vi "TirfModule.vi"() -> ()   [LabVIEW 2012]
doc: "DESCRIPTION:\nThe One-Axis Move (Accel - Max Velocity - Decel) VI completes a move to user-specified position on a single axis while using user-specified acceleration, maximum velocity, and deceleration values. It also provides a monitor to track the progress of the move.\n\n*Note: This VI can be used as a subVI in a higher level program.\n\nINSTRUCTIONS:\n(1) Be sure your board is initialized before running this VI. Refer to the Initialization topic in the FlexMotion VI Online Help, which can be launched by choosing FlexMotion VI Online Help in the Help menu.\n\n(2) Select the Board ID that corresponds to your FlexMotion controller in the Board Configuration Utility. \n\n(3) Select the axis number to be used.\n\n(4) Set the Target Position (in encoder counts) to which you want the axis to move.\n\n(5) Set the values you wish to use for maximum velocity (RPM), acceleration (RPS/S), and deceleration (RPS/S).\n\n(6) Run the VI.\n\nKEY PARAMETERS:\n(1) Target Position: The position to which you want to move. This value needs to be changed every time you run the VI. If you run the VI twice in a row with the same target position, the motor will not move the second time since it will already be at its target position.\n\n(2) Velocity: The maximum velocity for the specified axis during the move.\n\n(3) Acceleration: The acceleration for the axis during the move.\n\n(4) Deceleration: The deceleration for the axis during the move. (This may be different than the acceleration.)\n\nI/O CONNECTIONS OVERVIEW:\nThis example requires a system configuration with one axis."
uses:
  MicroDrive.dll
panel:
  out "Found Epi":bool
  in  "Axis":u16(ring)=6 items=["1"=1, "2"=2, "3"=3, "4"=4, "5"=5, "6"=6]
  in  "Load":bool
  in  "Save":bool
  in  "clear5":bool
  in  "clear4":bool
  in  "clear3":bool
  in  "clear2":bool
  in  "clear1":bool
  in  "clear all":bool
  in  "write 5":bool
  in  "write 4":bool
  in  "write 3":bool
  in  "write 2":bool
  in  "write 1":bool
  in  "p4":bool
  in  "p5":bool
  in  "p3":bool
  in  "p2":bool
  in  "p1":bool
  out "Cluster":cluster{"Name":string[], "Position":dbl[]}
  out "Array 2":string[](array[string])
  out "Array":dbl[](array[numeric])
  out "Moving":bool
  in  "EPI":bool
  in  "Store":bool
  out "Current Position":dbl
  in  "Direction:":bool=TRUE
  out "Device Handle":i32
  in  "Velocity (mm/s)":dbl=1.0 min=0.01 max=2.0 format="%.3f"
  in  "Move size (µm)":dbl=50.0 format="%.3f"
  out "Forward Limit":bool
  out "Reverse Limit":bool
  in  "stop":bool
  in  "Move":bool
  # "Move To:"
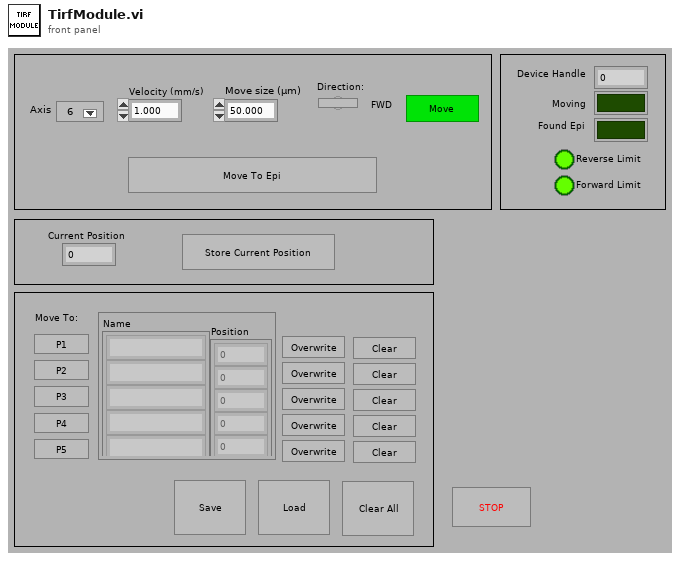
[diagram p1: front panel]
types:
  T1 = enum8{"Enabled", "Disabled", "Disabled and Grayed Out"}
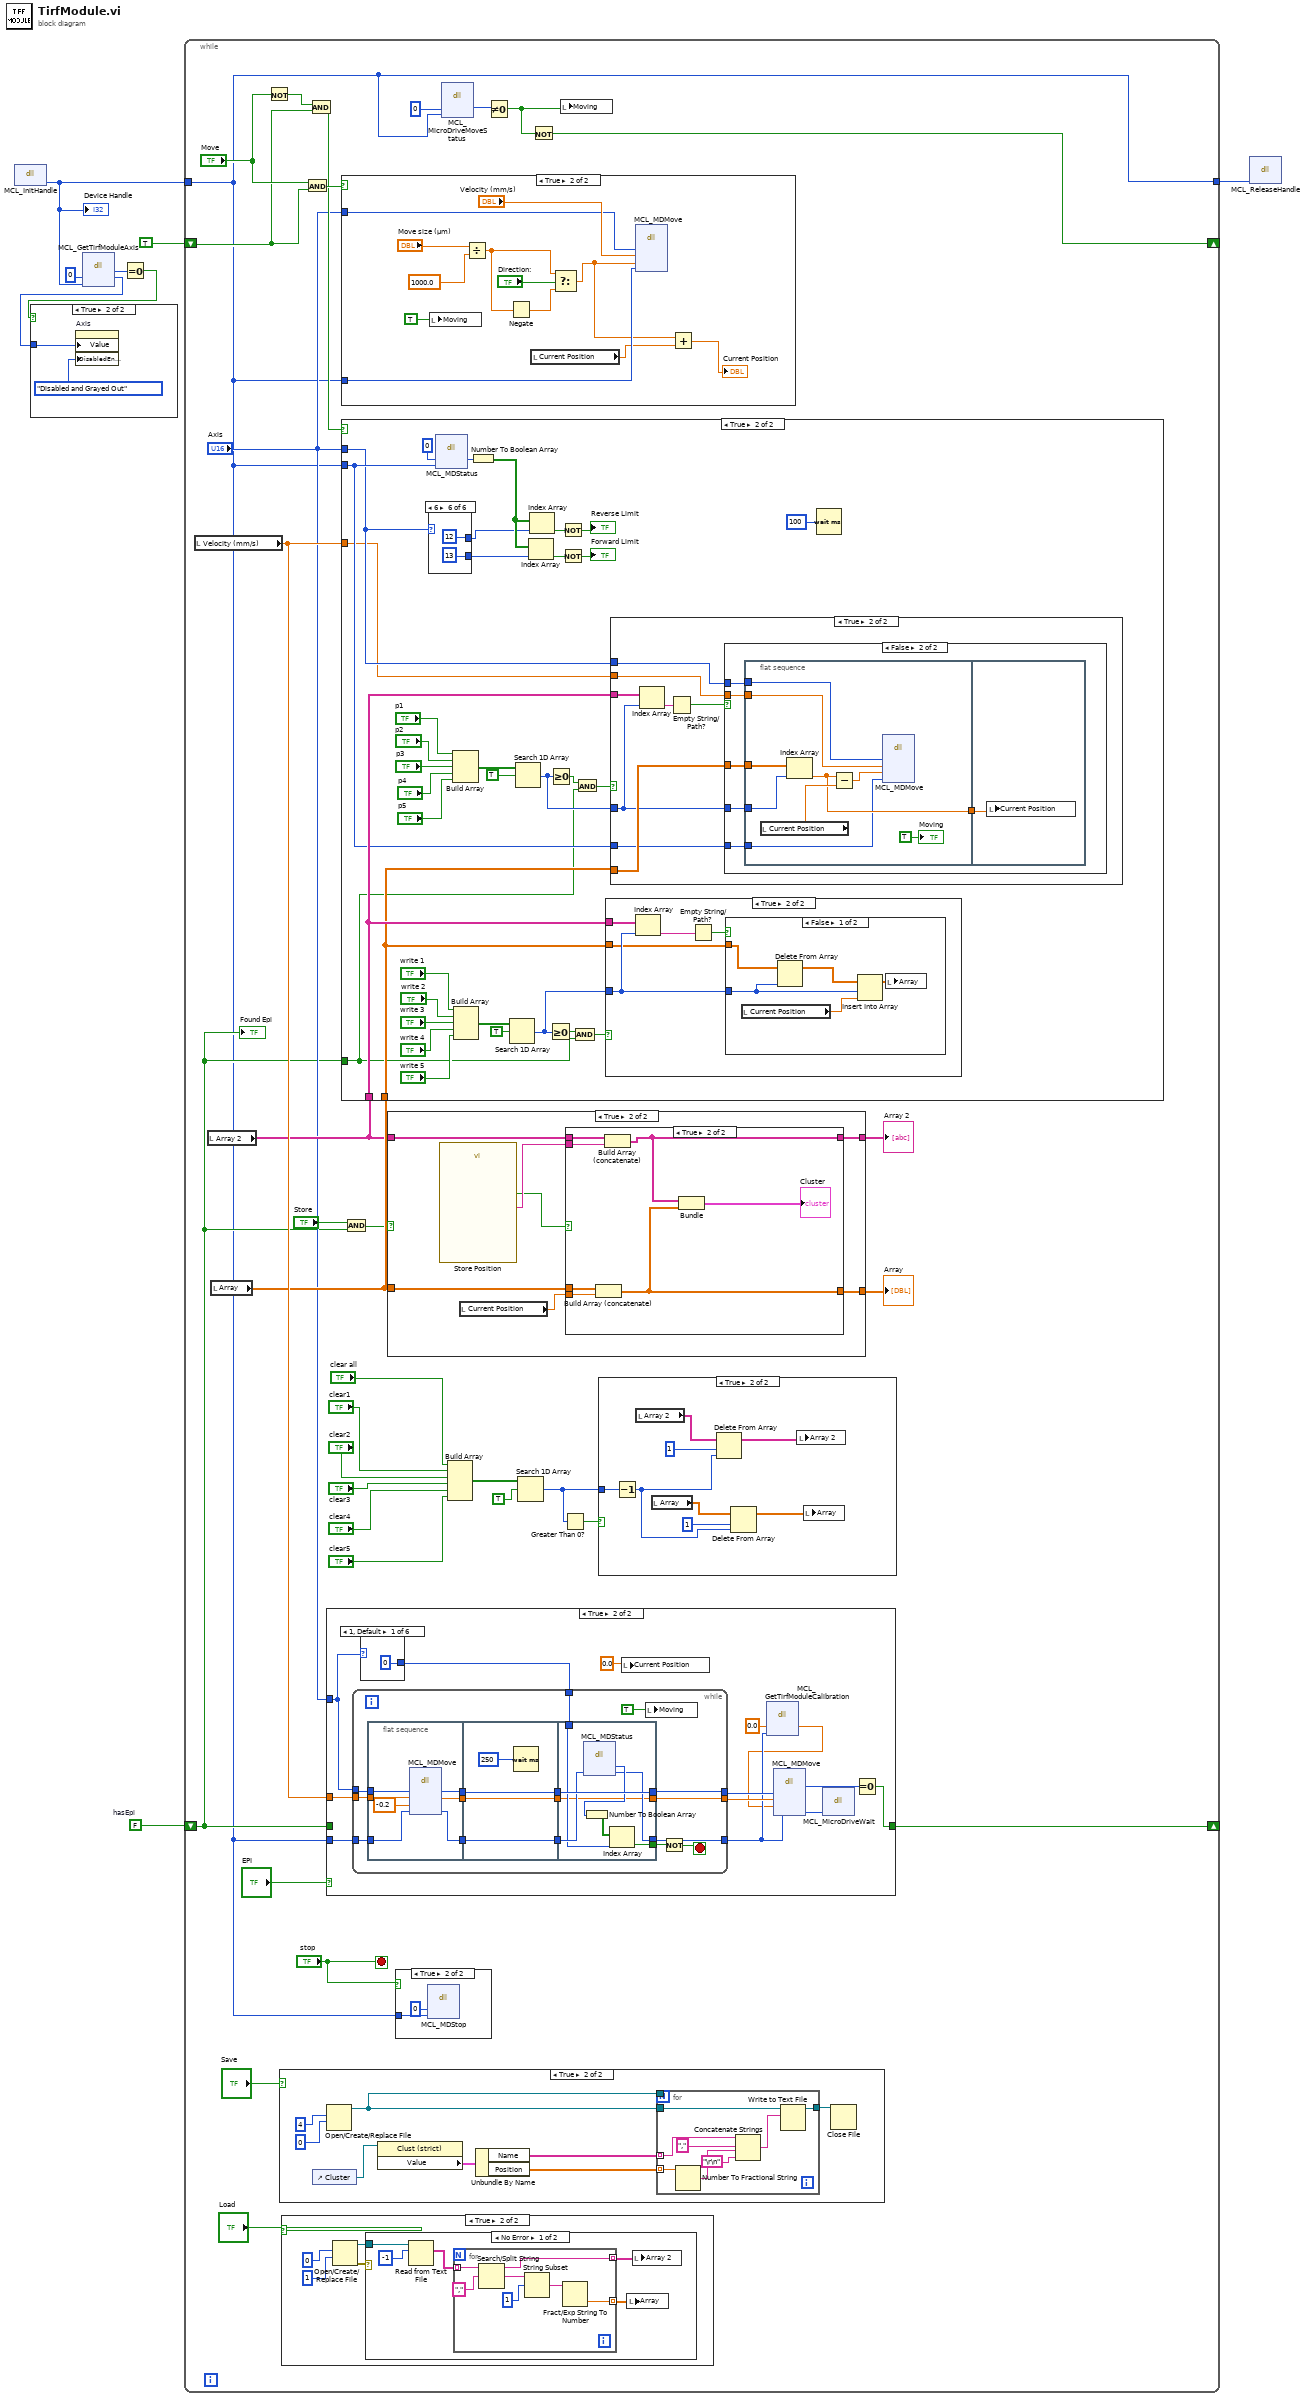
[diagram p0: block diagram]
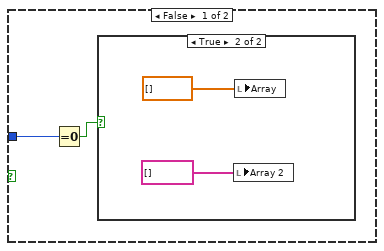
[diagram p6: hidden frame]
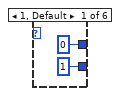
[diagram p9: hidden frame]
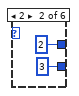
[diagram p10: hidden frame]
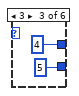
[diagram p11: hidden frame]
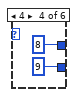
[diagram p12: hidden frame]
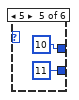
[diagram p13: hidden frame]
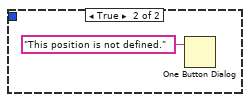
[diagram p15: hidden frame]
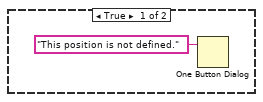
[diagram p17: hidden frame]
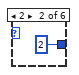
[diagram p19: hidden frame]
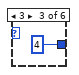
[diagram p20: hidden frame]
diagram:
  w6 = FALSE  # hasEpi
  n1 = dll-call lib="C:/Users/Labview/Desktop/TirfModule/MicroDrive.dll" fn="MCL_InitHandle"() -> ("return type"=w5:i32)  [unwired: 3 in, 2 out]
  "Device Handle" <- w5
  n2 = dll-call lib="C:/Users/Labview/Desktop/TirfModule/MicroDrive.dll" fn="MCL_GetTirfModuleAxis"("axis"=u16 0, "handle"=w5) -> ("return type"=w2:i32, "axis"=w3:i32)  [unwired: 4 in, 2 out]
  n3 = Equal To 0?(x=w2) -> (x = 0?=w1:bool)
  n4 = case shown="True" w1 {
    tunnel: w3 -> [_ w10]
    frame False {
    }
    frame True {
      n5 = property on="Axis" class="Ring (strict)"("Value"=w10, "DisabledEnum"=T1."Disabled and Grayed Out" ("Disabled")) -> ()  [unwired: 2 in, 2 out]
    }
  }
  n6 = while {
    tunnel: w5 -> [w13]
    shift-right: [w11] -> _
    shift-left: TRUE -> [w42]
    tunnel: [w13] -> w7
    shift-right: [w20] -> _
    shift-left: w6 -> [w16]
    stop <- "stop" stop-if-true
    n7 = local read "Velocity (mm/s)"() -> (w39:dbl)
    n8 = local read "Array 2"() -> (w35:string[])
    n9 = local read "Array"() -> (w38:dbl[])
    n10 = Not(x="Move") -> (.not. x?=w43:bool)
    n11 = case shown="True" "Save" {
      frame False {
      }
      frame True {
        n12 = control-ref of="Cluster"() -> (w68:refnum<vi>)
        n13 = Open/Create/Replace File(operation (0:open)=4, access (0:read/write)=0) -> (refnum out=w62:refnum<file>)  [unwired: 4 in, 2 out]
        n14 = property class="Clust (strict)"(reference=w68) -> ("Value"=w67:cluster{"Name":string[], "Position":dbl[]})  [unwired: 1 in, 2 out]
        n15 = Unbundle By Name(w67) -> ("Name"=w63:string[], "Position"=w61:dbl[])
        n16 = for {
          tunnel: w61 -> [w75] mode=indexing
          tunnel: w62 -> [_]
          tunnel: [w76] -> w64
          tunnel: w63 -> [w70] mode=indexing
          tunnel: w62 -> [w69]
          n17 = Number To Fractional String(number=w75) -> (F-format string=w71:string)  [unwired: 3 in]
          n18 = Concatenate Strings(w70, ",", w71, "\r\n") -> (w73:string)
          n19 = Write to Text File(file (use dialog)=w69, text=w73) -> (refnum out=w76:refnum<file>)  [unwired: 2 in, 2 out]
        }
        n20 = Close File(refnum=w64) -> ()  [unwired: 1 in, 2 out]
      }
    }
    n21 = case shown="True" "Load" {
      frame False {
      }
      frame True {
        n22 = Open/Create/Replace File(operation (0:open)=0, access (0:read/write)=1) -> (refnum out=w45:refnum<file>, error out=w46:errorcluster)  [unwired: 4 in, 1 out]
        n23 = case shown="No Error" w46 {
          tunnel: w45 -> [w53 _]
          frame No Error {
            n24 = Read from Text File(file (use dialog)=w53, count=-1) -> (text=w51:string[])  [unwired: 2 in, 3 out]
            n25 = for {
              tunnel: w51 -> [w60] mode=indexing
              tunnel: [w58] -> w50 mode=indexing
              tunnel: [w54] -> w49 mode=indexing
              n26 = Search/Split String(string=w60, search string/char (-)=",") -> (substring before match=w58:string, match + rest of string=w57:string)  [unwired: 1 in, 1 out]
              n27 = String Subset(string=w57, offset (0)=1) -> (substring=w55:string)  [unwired: 1 in]
              n28 = Fract/Exp String To Number(string=w55) -> (number=w54:dbl)  [unwired: 3 in, 1 out]
            }
            n29 = local write "Array"(w49) -> ()
            n30 = local write "Array 2"(w50) -> ()
          }
          frame Error {
          }
        }
      }
    }
    n31 = And(x="Move", y=w42) -> (x .and. y?=w41:bool)
    n32 = And(x=w43, y=w42) -> (x .and. y?=w37:bool)
    n33 = case shown="True" "EPI" {
      tunnel: w39 -> [_ w186]
      tunnel: w13 -> [_ w185]
      tunnel: "Axis" -> [_ w181]
      tunnel: w16 -> [w173 _]
      tunnel: [w173 w174] -> w20
      frame False {
      }
      frame True {
        n34 = case shown="1, Default" w181 {
          tunnel: [0 2 4 8 10 12] -> w180
          frame 1, Default {
          }
          frame 2 {
          }
          frame 3 {
          }
          frame 4 {
          }
          frame 5 {
          }
          frame 6 {
          }
        }
        n35 = while {
          tunnel: w186 -> [w208]
          tunnel: w185 -> [w204]
          tunnel: [w203] -> w177
          tunnel: w181 -> [w206]
          tunnel: [w205] -> w184
          tunnel: w180 -> [w198]
          tunnel: [w194] -> w179
          stop <- w207 stop-if-true
          n36 = flat-sequence {
            tunnel: w208 -> [w215]
            tunnel: w206 -> [w213]
            tunnel: w204 -> [w211]
            tunnel: [w212] -> w202
            tunnel: [w210] -> w201
            tunnel: [w209] -> w196
            tunnel: w202 -> [w219]
            tunnel: w201 -> [w218]
            tunnel: [w219] -> w200
            tunnel: [w218] -> w199
            tunnel: w196 -> [w216]
            tunnel: [w216] -> w195
            tunnel: [w223] -> w203
            tunnel: [w227] -> w205
            tunnel: w200 -> [w227]
            tunnel: w199 -> [w224]
            tunnel: w198 -> [w222]
            tunnel: [w221] -> w197
            tunnel: w195 -> [w220]
            tunnel: [w220] -> w194
            frame #0 {
              n37 = dll-call lib="C:/Users/Labview/Desktop/TirfModule/MicroDrive.dll" fn="MCL_MDMove"("axis"=w213, "velocity"=w215, "distance"=-0.2, "handle"=w211) -> ("axis"=w212:i32, "velocity"=w209:dbl, "handle"=w210:i32)  [unwired: 4 in, 3 out]
            }
            frame #1 {
              n38 = Wait (ms)(milliseconds to wait=u32 250) -> ()  [unwired: 1 out]
            }
            frame #2 {
              n39 = dll-call lib="C:/Users/Labview/Desktop/TirfModule/MicroDrive.dll" fn="MCL_MDStatus"("handle"=w224) -> ("status"=w226:u16, "handle"=w223:i32)  [unwired: 3 in, 4 out]
              n40 = Number To Boolean Array(number=w226) -> (Boolean array=w225:bool[])
              n41 = Index Array(array=w225, index=w222) -> (element=w221:bool)
            }
          }
          n42 = local write "Moving"(TRUE ("is Moving")) -> ()
          n43 = Not(x=w197) -> (.not. x?=w207:bool)
        }
        n44 = local write "Current Position"(0.0) -> ()
        n45 = dll-call lib="C:/Users/Labview/Desktop/TirfModule/MicroDrive.dll" fn="MCL_GetTirfModuleCalibration"("calMM"=0.0 ("distance"), "handle"=w177) -> ("calMM"=w176:dbl)  [unwired: 4 in, 3 out]
        n46 = dll-call lib="C:/Users/Labview/Desktop/TirfModule/MicroDrive.dll" fn="MCL_MDMove"("axis"=w184, "velocity"=w179, "distance"=w176, "handle"=w177) -> ("return type"=w175:i32, "handle"=w182:i32)  [unwired: 5 in, 3 out]
        n47 = dll-call lib="C:/Users/Labview/Desktop/TirfModule/MicroDrive.dll" fn="MCL_MicroDriveWait"("handle"=w182) -> ()  [unwired: 4 in, 3 out]
        n48 = Equal To 0?(x=w175) -> (x = 0?=w174:bool)
      }
    }
    n49 = case shown="True" w41 {
      tunnel: w13 -> [_ w257]
      tunnel: "Axis" -> [_ w249]
      frame False {
      }
      frame True {
        n50 = local write "Moving"(TRUE ("is Moving")) -> ()
        n51 = Divide(x="Move size (µm)", y=1000.0) -> (x/y=w254:dbl)
        n52 = Negate(x=w254) -> (-x=w255:dbl)
        n53 = local read "Current Position"() -> (w251:dbl)
        n54 = Select(t=w254, s="Direction:", f=w255) -> (s? t:f=w253:dbl)
        n55 = dll-call lib="C:/Users/Labview/Desktop/TirfModule/MicroDrive.dll" fn="MCL_MDMove"("axis"=w249, "velocity"="Velocity (mm/s)", "distance"=w253, "handle"=w257) -> ()  [unwired: 6 in, 4 out]
        n56 = Add(x=w253, y=w251) -> (x+y=→"Current Position":dbl)
      }
    }
    n57 = case shown="True" w37 {
      tunnel: w35 -> [_ w124]
      tunnel: w39 -> [_ w94]
      tunnel: w38 -> [_ w123]
      tunnel: "Axis" -> [_ w95]
      tunnel: w13 -> [_ w96]
      tunnel: w16 -> [_ w90]
      frame False {
      }
      frame True {
        n58 = case shown="6" w95 {
          tunnel: [0 2 4 8 10 12] -> w98
          tunnel: [1 3 5 9 11 13] -> w97
          frame 1, Default {
          }
          frame 2 {
          }
          frame 3 {
          }
          frame 4 {
          }
          frame 5 {
          }
          frame 6 {
          }
        }
        n59 = dll-call lib="C:/Users/Labview/Desktop/TirfModule/MicroDrive.dll" fn="MCL_MDStatus"("status"=u16 0, "handle"=w96) -> ("status"=w120:u16)  [unwired: 4 in, 3 out]
        n60 = Build Array("p1", "p2", "p3", "p4", "p5") -> (w105:bool[])
        n61 = Build Array("write 1", "write 2", "write 3", "write 4", "write 5") -> (w113:bool[])
        n62 = Number To Boolean Array(number=w120) -> (Boolean array=w119:bool[])
        n63 = Search 1D Array(1D array=w113, element=TRUE) -> (index of element=w112:i32)  [unwired: 1 in]
        n64 = Search 1D Array(1D array=w105, element=TRUE) -> (index of element=w99:i32)  [unwired: 1 in]
        n65 = Index Array(array=w119, index=w97) -> (element=w118:bool)
        n66 = Index Array(array=w119, index=w98) -> (element=w117:bool)
        n67 = Greater Or Equal To 0?(x=w112) -> (x >= 0?=w93:bool)
        n68 = Greater Or Equal To 0?(x=w99) -> (x >= 0?=w89:bool)
        n69 = Not(x=w117) -> (.not. x?=→"Reverse Limit":bool)
        n70 = Not(x=w118) -> (.not. x?=→"Forward Limit":bool)
        n71 = And(x=w93, y=w90) -> (x .and. y?=w92:bool)
        n72 = And(x=w89, y=w90) -> (x .and. y?=w91:bool)
        n73 = case shown="True" w92 {
          tunnel: w124 -> [_ w141]
          tunnel: w123 -> [_ w137]
          tunnel: w112 -> [_ w138]
          frame False {
          }
          frame True {
            n74 = Index Array(array=w141, index=w138) -> (element=w140:string)
            n75 = Empty String/Path?(string/path=w140) -> (empty?=w139:bool)
            n76 = case shown="False" w139 {
              tunnel: w138 -> [w145 _]
              tunnel: w137 -> [w142 _]
              frame False {
                n77 = local read "Current Position"() -> (w144:dbl)
                n78 = Delete From Array(array=w142, index=w145) -> (array with subset deleted=w146:dbl[])  [unwired: 1 in, 1 out]
                n79 = Insert Into Array(array=w146, index=w145, new element=w144) -> (w143:dbl[])
                n80 = local write "Array"(w143) -> ()
              }
              frame True {
                n81 = One Button Dialog(message="This position is not defined.") -> ()  [unwired: 1 in, 1 out]
              }
            }
          }
        }
        n82 = case shown="True" w91 {
          tunnel: w123 -> [_ w155]
          tunnel: w96 -> [_ w154]
          tunnel: w94 -> [_ w153]
          tunnel: w124 -> [_ w152]
          tunnel: w99 -> [_ w149]
          tunnel: w95 -> [_ w148]
          frame False {
          }
          frame True {
            n83 = Index Array(array=w152, index=w149) -> (element=w151:string)
            n84 = Empty String/Path?(string/path=w151) -> (empty?=w150:bool)
            n85 = case shown="False" w150 {
              tunnel: w155 -> [_ w162]
              tunnel: w154 -> [_ w161]
              tunnel: w153 -> [_ w160]
              tunnel: w149 -> [_ w159]
              tunnel: w148 -> [_ w157]
              frame True {
                n86 = One Button Dialog(message="This position is not defined.") -> ()  [unwired: 1 in, 1 out]
              }
              frame False {
                n87 = flat-sequence {
                  tunnel: w162 -> [w171]
                  tunnel: w161 -> [w165]
                  tunnel: w160 -> [w164]
                  tunnel: w159 -> [w168]
                  tunnel: [w166] -> w158
                  tunnel: w157 -> [w163]
                  tunnel: w158 -> [w172]
                  frame #0 {
                    n88 = local read "Current Position"() -> (w169:dbl)
                    n89 = Index Array(array=w171, index=w168) -> (element=w166:dbl)
                    n90 = Subtract(x=w166, y=w169) -> (x-y=w170:dbl)
                    n91 = dll-call lib="C:/Users/Labview/Desktop/TirfModule/MicroDrive.dll" fn="MCL_MDMove"("axis"=w163, "velocity"=w164, "distance"=w170, "handle"=w165) -> ()  [unwired: 6 in, 4 out]
                    "Moving" <- TRUE ("is Moving")
                  }
                  frame #1 {
                    n92 = local write "Current Position"(w172) -> ()
                  }
                }
              }
            }
          }
        }
        n93 = Wait (ms)(milliseconds to wait=100) -> ()  [unwired: 1 out]
      }
    }
    n94 = And(x="Store", y=w16) -> (x .and. y?=w17:bool)
    n95 = case shown="True" w17 {
      tunnel: w35 -> [w230 w237]
      tunnel: [w230 w233] -> w34
      tunnel: w38 -> [w228 w236]
      tunnel: [w228 w232] -> w36
      frame False {
        n96 = Bundle("Array 2"=w230, "Array"=w228) -> (w229:cluster{"Array 2":string[], "Array":dbl[]})  [unwired: 1 in]
        n97 = local write "Cluster"(w229) -> ()
      }
      frame True {
        n98 = call "Store Position"() -> ("Name"=w235:string, "OK"=w231:bool)  [unwired: 17 in, 1 out]
        n99 = local read "Current Position"() -> (w234:dbl)
        n100 = case shown="True" w231 {
          tunnel: w237 -> [w239 w246]
          tunnel: w236 -> [w238 w245]
          tunnel: w235 -> [_ w244]
          tunnel: w234 -> [_ w243]
          tunnel: [w239 w242] -> w233
          tunnel: [w238 w240] -> w232
          frame False {
          }
          frame True {
            n101 = Build Array (concatenate)(w245, w243) -> (w240:dbl[])
            n102 = Build Array (concatenate)(w246, w244) -> (w242:string[])
            n103 = Bundle(w242, w240) -> (→"Cluster":cluster{string[], dbl[]})  [unwired: 1 in]
          }
        }
      }
    }
    "Array" <- w36
    "Array 2" <- w34
    n104 = case shown="True" "stop" {
      tunnel: w13 -> [_ w247]
      frame False {
      }
      frame True {
        n105 = dll-call lib="C:/Users/Labview/Desktop/TirfModule/MicroDrive.dll" fn="MCL_MDStop"("status"=0, "handle"=w247) -> ()  [unwired: 4 in, 4 out]
      }
    }
    n106 = dll-call lib="C:/Users/Labview/Desktop/TirfModule/MicroDrive.dll" fn="MCL_MicroDriveMoveStatus"("isMoving"=0 ("length"), "handle"=w13) -> ("isMoving"=w14:i32)  [unwired: 4 in, 3 out]
    n107 = Build Array("clear all", "clear1", "clear2", "clear3", "clear4", "clear5") -> (w27:bool[])
    n108 = Not Equal To 0?(x=w14) -> (x != 0?=w12:bool)
    n109 = Search 1D Array(1D array=w27, element=TRUE) -> (index of element=w26:i32)  [unwired: 1 in]
    n110 = Not(x=w12) -> (.not. x?=w11:bool)
    n111 = local write "Moving"(w12) -> ()
    n112 = Greater Than 0?(x=w26) -> (x > 0?=w28:bool)
    n113 = case shown="True" w28 {
      tunnel: w26 -> [w78 w84]
      frame False {
        n114 = Equal To 0?(x=w78) -> (x = 0?=w77:bool)
        n115 = case shown="True" w77 {
          frame False {
          }
          frame True {
            n116 = local write "Array 2"(string[] []) -> ()
            n117 = local write "Array"(dbl[] []) -> ()
          }
        }
      }
      frame True {
        n118 = Decrement(x=w84) -> (x-1=w81:i32)
        n119 = local read "Array 2"() -> (w86:string[])
        n120 = local read "Array"() -> (w85:dbl[])
        n121 = Delete From Array(array=w86, length=1, index=w81) -> (array with subset deleted=w83:string[])  [unwired: 1 out]
        n122 = Delete From Array(array=w85, length=1, index=w81) -> (array with subset deleted=w82:dbl[])  [unwired: 1 out]
        n123 = local write "Array 2"(w83) -> ()
        n124 = local write "Array"(w82) -> ()
      }
    }
    "Found Epi" <- w16
  }
  n125 = dll-call lib="C:/Users/Labview/Desktop/TirfModule/MicroDrive.dll" fn="MCL_ReleaseHandle"("handle"=w7) -> ()  [unwired: 4 in, 3 out]
